vi "Tick Period to RPM.vi"(8 "Tire Diameter(m)":fxp<+,16,1>, 10 "Tick Period":u32) -> (0 "vWheel":fxp<+/-,32,18>, 2 "nWheel":fxp<+/-,29,16>)   [LabVIEW 2015]
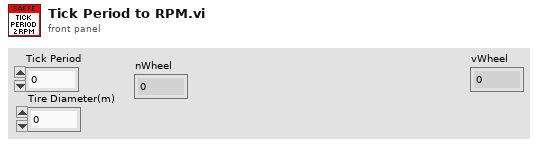
[diagram p1: front panel]
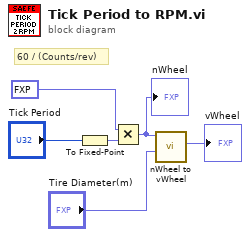
[diagram p0: block diagram]
diagram:
  # "60 / (Counts/rev)"
  n1 = To Fixed-Point(number="Tick Period") -> (fixed-point=w2:fxp<+,32,16>)  [unwired: 1 in]
  n2 = Multiply(x=fxp<+,1,-1> 0.25, y=w2) -> (x*y=w1:fxp<+/-,29,16>)
  "nWheel" <- w1
  n3 = call "nWheel to vWheel.vi"("Tire Diameter(m)"="Tire Diameter(m)", "nWheel"=w1) -> ("vWheel"=→"vWheel":fxp<+/-,32,18>)  [unwired: 9 in]
